vi "Timer.vi"(1 "Seconds (string)":string) -> (0 "Done":bool)   [LabVIEW 2017, in "Apple script.lvlib"]
doc: "A timer. Converts a string parameter into a number to be used as the time."
uses:
  Apple script.lvlib
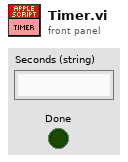
[diagram p1: front panel]
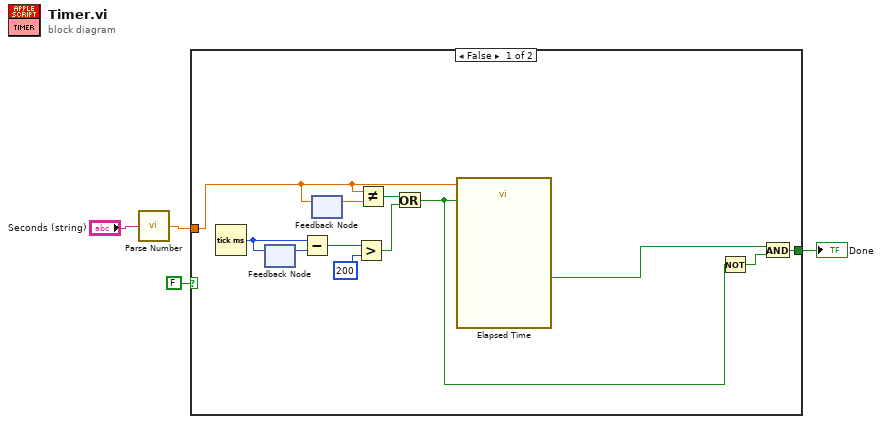
[diagram p0: block diagram]
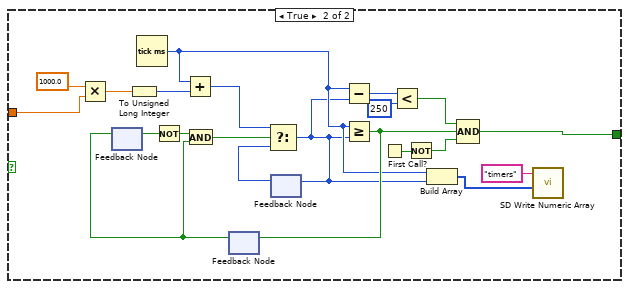
[diagram p2: hidden frame]
diagram:
  n1 = call "Parse Number.vi"("String"="Seconds (string)") -> ("Number"=w2:dbl)
  n2 = case shown="False" FALSE {
    tunnel: [w14 w23] -> w4
    tunnel: w2 -> [w12 w22]
    frame False {
      n3 = Tick Count (ms)() -> (millisecond timer value=w8:u32)
      n4 = feedback #1() -> (w7:u32)  [unwired: 1 in]
      n5 = feedback-in #1(w8) -> ()
      n6 = Subtract(x=w8, y=w7) -> (x-y=w9:u32)
      n7 = feedback #2() -> (w13:dbl)  [unwired: 1 in]
      n8 = feedback-in #2(w12) -> ()
      n9 = Greater?(x=w9, y=u32 200) -> (0:w5:bool)
      n10 = Not Equal?(x=w12, y=w13) -> (x != y?=w11:bool)
      n11 = Or(x=w11, y=w5) -> (x .or. y?=w10:bool)
      n12 = call "Elapsed Time"("Time Target (s)"=w12, "Reset"=w10) -> ("Time has Elapsed"=w16:bool)  [unwired: 10 in, 7 out]
      n13 = Not(x=w10) -> (.not. x?=w15:bool)
      n14 = And(x=w16, y=w15) -> (x .and. y?=w14:bool)
    }
    frame True {
      n15 = Multiply(x=1000.0, y=w22) -> (x*y=w31:dbl)
      n16 = feedback #3() -> (w34:bool)  [unwired: 1 in]
      n17 = To Unsigned Long Integer(number=w31) -> (unsigned 32bit integer=w30:u32)
      n18 = Tick Count (ms)() -> (millisecond timer value=w20:u32)
      n19 = Not(x=w34) -> (.not. x?=w33:bool)
      n20 = Add(x=w20, y=w30) -> (x+y=w37:u32)
      n21 = feedback #4() -> (w29:bool)  [unwired: 1 in]
      n22 = feedback-in #3(w29) -> ()
      n23 = And(x=w33, y=w29) -> (x .and. y?=w35:bool)
      n24 = feedback #5() -> (w36:u32)  [unwired: 1 in]
      n25 = Select(t=w37, s=w35, f=w36) -> (s? t:f=w19:u32)
      n26 = feedback-in #5(w19) -> ()
      n27 = Subtract(x=w20, y=w19) -> (x-y=w27:u32)
      n28 = Greater Or Equal?(x=w20, y=w19) -> (x >= y?=w25:bool)
      n29 = feedback-in #4(w25) -> ()
      n30 = First Call?() -> (First Call?: T/F=w28:bool)
      n31 = Less?(x=w27, y=u32 250) -> (x < y?=w24:bool)
      n32 = Not(x=w28) -> (.not. x?=w21:bool)
      n33 = Build Array(w20, w19) -> (w18:u32[])
      n34 = Compound Arithmetic op=AND(w24, w25, w21) -> (w23:bool)
      n35 = call <vilib>:"SD Write Numeric Array.vi"("Numeric Array"=w18, "Name"="timers") -> ()  [unwired: 8 in, 2 out]
    }
  }
  "Done" <- w4
